vi "reset.vi"(8 "error in (no error)":errorcluster, 11 "ScopeKeysight in":refnum<class "ScopeKeysight.lvclass">) -> (0 "error out":errorcluster, 3 "ScopeKeysight out":refnum<class "ScopeKeysight.lvclass">)   [LabVIEW 2023, in "ScopeKeysight.lvclass"]
doc: "Reset the instrument to default/factory settings."
uses:
  ScopeKeysight.lvclass
  ScopeKeysight.lvclass/ScopeKeysight.ctl
  Scope.lvclass
  Driver/Keysight-DSQx3014T.lvlib
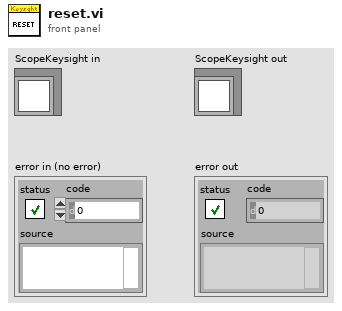
[diagram p1: front panel]
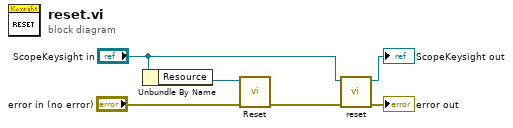
[diagram p0: block diagram]
diagram:
  n1 = Unbundle By Name("ScopeKeysight in") -> ("Resource"=w3:refnum<visa-resource-name>)
  n2 = call "Reset.vi"("error in (no error)"="error in (no error)", "VISA resource name"=w3) -> ("error out"=w1:errorcluster)  [unwired: 8 in, 1 out]
  n3 = call-parent "reset.vi"("error in (no error)"=w1, "Instrument in"="ScopeKeysight in") -> ("error out"=→"error out":errorcluster, "Instrument out"=→"ScopeKeysight out":refnum<class "ScopeKeysight.lvclass">)  [unwired: 8 in]
